vi "Read currentBallZone.vi"(8 "error in (no error)":errorcluster, 11 "Ally in":refnum<class "Ally.lvclass">) -> (0 "error out":errorcluster, 2 "Enum":T1, 3 "Ally out":refnum<class "Ally.lvclass">)   [LabVIEW 2023, in "Ally.lvclass"]
uses:
  Ally.lvclass
  Zone_class/zones.ctl
  Ally.lvclass/Ally.ctl
  Zone_class/Zone.lvclass
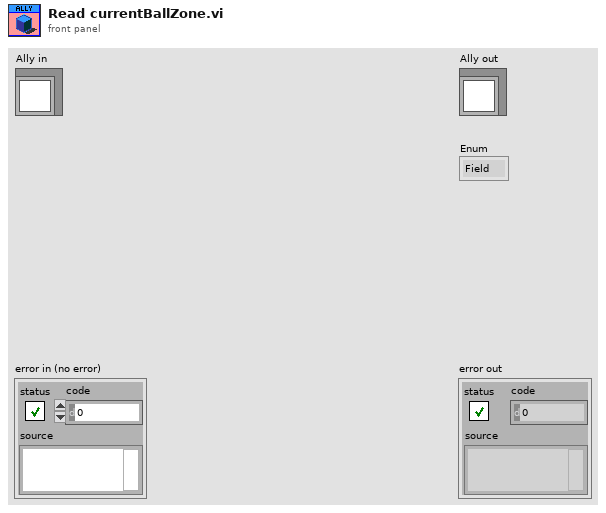
[diagram p1: front panel]
types:
  T1 = typedef "Zone.lvclass/zones.ctl" = enum16{"Field", "LeftSide", "RightSide", "MidField", "LeftForward", "RightForward", "LeftMidField", "RightMidField", "LeftWing", "CenterForward", "RightWing", "Size"}
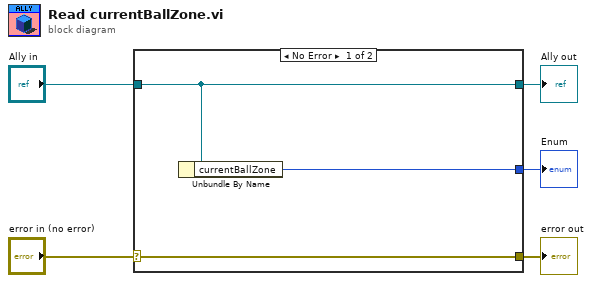
[diagram p0: block diagram]
diagram:
  n1 = case shown="No Error" "error in (no error)" {
    selector: "error in (no error)" -> [w8 w9]
    tunnel: [w8 w9] -> w4
    tunnel: [w7 w10] -> w2
    tunnel: "Ally in" -> [w7 w10]
    tunnel: [w6 _] -> w1
    frame No Error {
      n2 = Unbundle By Name(w7) -> ("currentBallZone"=w6:T1)
    }
    frame Error {
    }
  }
  "error out" <- w4
  "Ally out" <- w2
  "Enum" <- w1
